vi "1_SimpleDemo_HHHisto.vi"() -> ()   [LabVIEW 2010]
uses:
  _lib/PQ/HydraHarp/hhlib_x86_x64_UIThread.llb/HH_DllPath_global.vi
  _lib/PQ/HydraHarp/HH_MeasMode.ctl
  _lib/PQ/HydraHarp/HH_RefSource.ctl
  _lib/PQ/HydraHarp/HH_LibVersion_global.vi
panel:
  in  "Binning":i32(ring) caption="Resolution [ps]" items=["1", "2", "4", "8", "16", "32", "64", "128", "256", "512", "1024", "2048", "4096", "8192", "16384", "32768", "65536", "131072", "262144", "524288", "1048576", "2097152", "4194304", "8388608", "16777216", "33554432"]
  in  "HistoLength":i32(ring)=6 caption="Histo Length" items=["1024", "2048", "4096", "8192", "16384", "32768", "65536"]
  in  "Acqu.Time":i32=10000 caption="Acqu.Time [ms]" min=1 max=360000000 step=1
  in  "GlobalOffset":i32 caption="GlobalOffset [ns]" min=0 max=500000 step=1
  in  "OverflowLevel":u32=65535 min=1 step=1
  in  "StopOnOverflow":bool=TRUE
  in  "InputZeroX":i32=10 caption="ZeroCr. [mV]" min=0 max=40 step=1
  in  "InputCFDLevel":i32=50 caption="CFDLevel [mV]" min=0 max=1000 step=1
  in  "Offset":i32 caption="Offset [ps]" min=-99999 max=99999 step=1
  in  "Enable":bool=TRUE
  in  "SyncZeroX":i32=10 caption="ZeroCr. [mV]" min=0 max=40 step=1
  in  "SyncCFDLevel":i32=50 caption="CFDLevel [mV]" min=0 max=1000 step=1
  in  "SyncOffset":i32 caption="SyncOffset [ps]" min=-99999 max=99999 step=1
  in  "SyncDivider":i32(ring)=8 items=["1"=1, "2"=2, "4"=4, "8"=8, "16"=16]
  out "HistoGraph":T1(graph)={0.0, "Resolution"=0.08, "Histogram"=[]}
  out "CountRates":i32[](array[numeric]) caption="Count Rates [cps]"
  out "SyncRate":i32 caption="Sync Rate [cps]"
  in  "stop":bool
  out "error out":errorcluster
  # "Acquisition"
  # "All Channels"
  # "Sync"
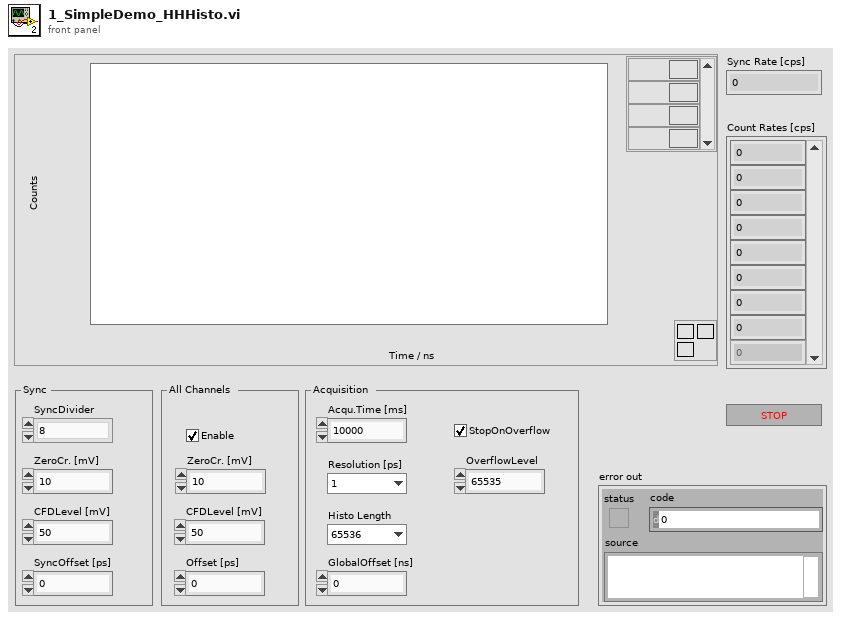
[diagram p1: front panel]
types:
  T1 = cluster{dbl, "Resolution":dbl, "Histogram":u32[][]}
  T2 = typedef "HH_MeasMode.ctl" = i32
  T3 = typedef "HH_RefSource.ctl" = enum16{"internal", "external"}
  T4 = typedef "HH_InitInfo.ctl" = cluster{"Library Version":string, "Serial No.":string, "Model":string, "Partnum":string, "Version":string, "features":i32, "nchannels":i32, "nummod":i32, "Model Codes":i32[], "Version Codes":i32[], "Base Resolution":dbl, "Bin Steps":i32}
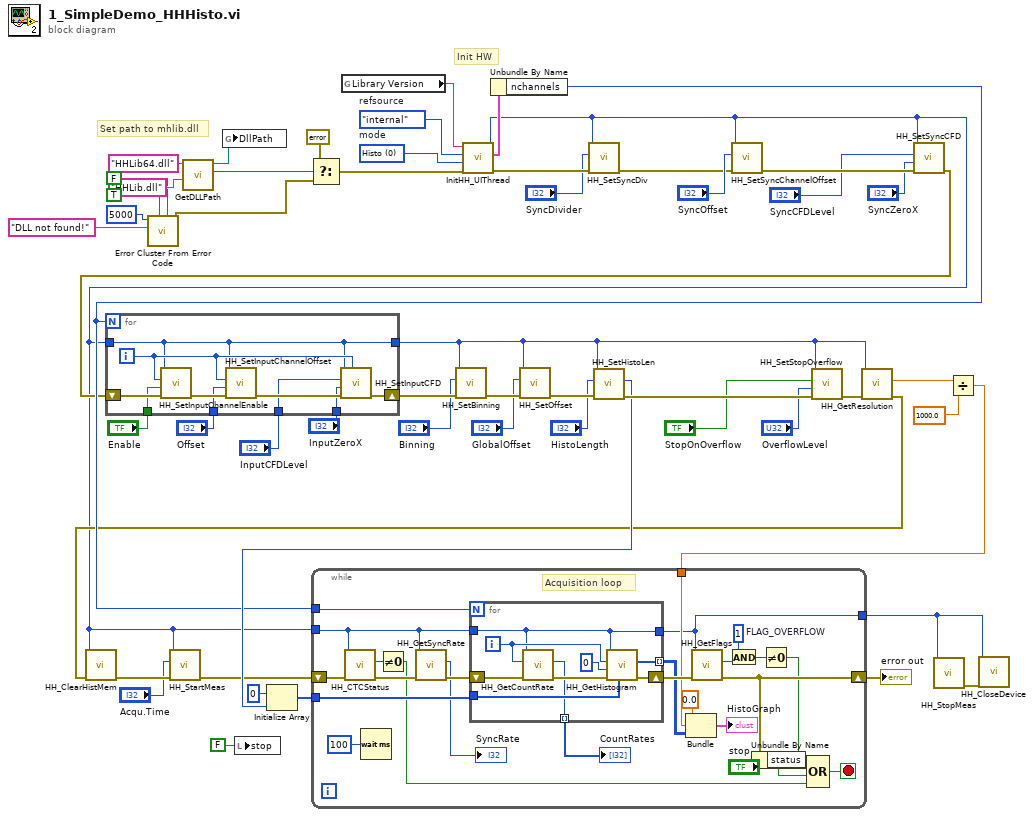
[diagram p0: block diagram]
diagram:
  w53 = T2 0 items=["Histo"=0, "T2"=2, "T3"=3, "Conti"=8]  # mode
  w54 = HH_RefSource."internal"  # refsource
  # "Init HW"
  # "Set path to mhlib.dll"
  n1 = call <vilib>:"Error Cluster From Error Code.vi"("is warning? (False)"=FALSE, "show call chain? (False)"=TRUE, "error message (\"\")"="DLL not found!" ("error message (\"\")"), "error code (0)"=5000) -> ("error out"=w52:errorcluster)  [unwired: 5 in]
  n2 = call "GetDLLPath.vi"("DllName_32bit"="HHLib.dll" ("name or relative path"), "DllName_64bit"="HHLib64.dll" ("name or relative path")) -> ("file exists?"=w50:bool, "DLLPath"=w49:path)  [unwired: 8 in]
  n3 = global write "HH_DllPath_global.vi" "DllPath"(w49) -> ()
  n4 = local write "stop"(FALSE ("stop")) -> ()
  n5 = Select(t=errorcluster {"status"=FALSE, "code"=0, "source"=""} ("error IO"), s=w50, f=w52) -> (s? t:f=w46:errorcluster)
  n6 = global read "HH_LibVersion_global.vi" "Library Version"() -> (w7:string)
  n7 = call "InitHH_UIThread.vi"("error in (no error)"=w46, "mode"=w53, "refsource"=w54, "Library Version"=w7) -> ("error out"=w40:errorcluster, "Init Info"=w42:T4, "DevIdx"=w13:i32)  [unwired: 5 in]
  n8 = Unbundle By Name(w42) -> ("nchannels"=w22:i32)
  n9 = call "HH_SetSyncDiv.vi"("error in (no error)"=w40, "SyncDivider"="SyncDivider", "devidx"=w13) -> ("error out"=w39:errorcluster)  [unwired: 7 in, 1 out]
  n10 = call "HH_SetSyncChannelOffset.vi"("error in (no error)"=w39, "Offset"="SyncOffset", "devidx"=w13) -> ("error out"=w44:errorcluster)  [unwired: 7 in, 1 out]
  n11 = call "HH_SetSyncCFD.vi"("error in (no error)"=w44, "CFD ZeroCross"="SyncZeroX", "CFD Level"="SyncCFDLevel", "devidx"=w13) -> ("error out"=w21:errorcluster)  [unwired: 6 in, 1 out]
  n12 = for {
    N: w22 -> [_]
    shift-right: [w61] -> w41
    shift-left: w21 -> [w64]
    tunnel: w13 -> [w59]
    tunnel: [w59] -> w16
    tunnel: "Enable" -> [w58]
    tunnel: "Offset" -> [w57]
    tunnel: "InputZeroX" -> [w56]
    tunnel: "InputCFDLevel" -> [w55]
    i -> [w60]
    n13 = call "HH_SetInputChannelEnable.vi"("error in (no error)"=w64, "enable"=w58, "channel"=w60, "devidx"=w59) -> ("error out"=w63:errorcluster)  [unwired: 6 in, 1 out]
    n14 = call "HH_SetInputChannelOffset.vi"("error in (no error)"=w63, "Offset"=w57, "channel"=w60, "devidx"=w59) -> ("error out"=w62:errorcluster)  [unwired: 6 in, 1 out]
    n15 = call "HH_SetInputCFD.vi"("CFD Channel"=w60, "error in (no error)"=w62, "CFD ZeroCross"=w56, "CFD Level"=w55, "devidx"=w59) -> ("error out"=w61:errorcluster)  [unwired: 5 in, 1 out]
  }
  n16 = call "HH_SetBinning.vi"("error in (no error)"=w41, "Binning"="Binning", "devidx"=w16) -> ("error out"=w37:errorcluster)  [unwired: 7 in, 1 out]
  n17 = call "HH_SetOffset.vi"("error in (no error)"=w37, "Offset"="GlobalOffset", "devidx"=w16) -> ("error out"=w35:errorcluster)  [unwired: 7 in, 1 out]
  n18 = call "HH_SetHistoLen.vi"("error in (no error)"=w35, "lencode"="HistoLength", "devidx"=w16) -> ("error out"=w34:errorcluster, "actuallen"=w27:i32)  [unwired: 6 in, 1 out]
  n19 = Initialize Array(u32 0, w27) -> (w26:u32[])
  n20 = call "HH_SetStopOverflow.vi"("error in (no error)"=w34, "stopcount"="OverflowLevel", "StopOnOverflow"="StopOnOverflow", "devidx"=w16) -> ("error out"=w17:errorcluster)  [unwired: 6 in, 1 out]
  n21 = call "HH_GetResolution.vi"("error in (no error)"=w17, "devidx"=w16) -> ("error out"=w14:errorcluster, "resolution"=w15:dbl)  [unwired: 7 in, 1 out]
  n22 = call "HH_ClearHistMem.vi"("error in (no error)"=w14, "devidx"=w13) -> ("error out"=w31:errorcluster)  [unwired: 8 in, 1 out]
  n23 = call "HH_StartMeas.vi"("error in (no error)"=w31, "tacq"="Acqu.Time", "devidx"=w13) -> ("error out"=w12:errorcluster)  [unwired: 7 in, 1 out]
  n24 = Divide(x=w15, y=1000.0) -> (x/y=w23:dbl)
  n25 = while {
    shift-right: [w77] -> w29
    shift-left: w12 -> [w88]
    tunnel: w13 -> [w84]
    tunnel: w22 -> [w87]
    tunnel: w26 -> [w79]
    tunnel: w23 -> [w71]
    tunnel: [w66] -> w6
    stop <- w78 stop-if-true
    w82 = 1  # FLAG_OVERFLOW
    # "Acquisition loop"
    n26 = call "HH_CTCStatus.vi"("error in (no error)"=w88, "devidx"=w84) -> ("error out"=w86:errorcluster, "ctcstatus"=w89:i32)  [unwired: 7 in, 1 out]
    n27 = Wait (ms)(milliseconds to wait=u32 100) -> ()  [unwired: 1 out]
    n28 = Not Equal To 0?(x=w89) -> (x != 0?=w68:bool)
    n29 = call "HH_GetSyncRate.vi"("error in (no error)"=w86, "devidx"=w84) -> ("error out"=w85:errorcluster, "syncrate"=→"SyncRate":i32)  [unwired: 7 in, 1 out]
    n30 = for {
      N: w87 -> [_]
      shift-right: [w98] -> w83
      shift-left: w85 -> [w96]
      tunnel: w84 -> [w93]
      tunnel: [w93] -> w66
      tunnel: w79 -> [w92]
      tunnel: [w91] -> w74 mode=indexing
      tunnel: [w90] -> w73 mode=indexing
      i -> [w94]
      n31 = call "HH_GetCountRate.vi"("error in (no error)"=w96, "Channel"=w94, "devidx"=w93) -> ("error out"=w95:errorcluster, "rate"=w91:i32)  [unwired: 6 in, 1 out]
      n32 = call "HH_GetHistogram.vi"("Chcount"=w92, "error in (no error)"=w95, "clear"=0, "channel"=w94, "devidx"=w93) -> ("error out"=w98:errorcluster, "Histogram"=w90:u32[])  [unwired: 4 in, 1 out]
    }
    "CountRates" <- w74
    n33 = Bundle(0.0, w71, "Histogram"=w73) -> (→"HistoGraph":cluster{dbl, dbl, "Histogram":u32[][]})  [unwired: 1 in]
    n34 = call "HH_GetFlags.vi"("error in (no error)"=w83, "devidx"=w66) -> ("error out"=w77:errorcluster, "flags"=w80:i32)  [unwired: 7 in, 1 out]
    n35 = And(x=w82, y=w80) -> (x .and. y?=w81:i32)
    n36 = Unbundle By Name(w77) -> ("status"=w65:bool)
    n37 = Not Equal To 0?(x=w81) -> (x != 0?=w76:bool)
    n38 = Compound Arithmetic op=OR(w65, w76, "stop", w68) -> (w78:bool)
  }
  "error out" <- w29
  n39 = call "HH_StopMeas.vi"("devidx"=w6) -> ("error out"=w5:errorcluster)  [unwired: 9 in, 1 out]
  n40 = call "HH_CloseDevice.vi"("error in (no error)"=w5, "devidx"=w6) -> ()  [unwired: 8 in, 2 out]
